vi "Shift_Value_CH0_calibration_Rev02x.vi"(0 "IN1 Shift Val1":dbl, 1 "Enable memory wright":bool, 3 "Range IN1":dbl, 4 "USB Interface Name":refnum<visa-resource-name>="COM3", 5 "Input buffer size":u32=16384, 7 "error in (no error)":errorcluster, 13 "WRITE":bool, 27 "Sign Value":dbl) -> (8 "MB address":string, 9 "MB value":u8 format="%x", 12 "UB address":string, 14 "HB address":string, 15 "error out":errorcluster, 16 "LB address":string, 17 "UB value":u8 format="%x", 19 "Data string CH0":string, 20 "IN1 shift uV":dbl, 21 "IN1 shift  HEX uV":u32 format="%x", 23 "Sign Addrss":string, 24 "HB value":u8 format="%x", 25 "LB value":u8 format="%x")   [LabVIEW 2012]
panel:
  out "LB value":string
  out "HB value":string
  out "UB value":string
  out "MB value":string
  # "1. Computes address based on the input range \"Range IN\"\n2. Take absolute values of positive and negative voltage reads in uV compares them and subtracts smaller value from the larger one. The result is devided by 2.\nIf VAL1>VAL2: ( |VAL1| - |VAL2| )/ 2"
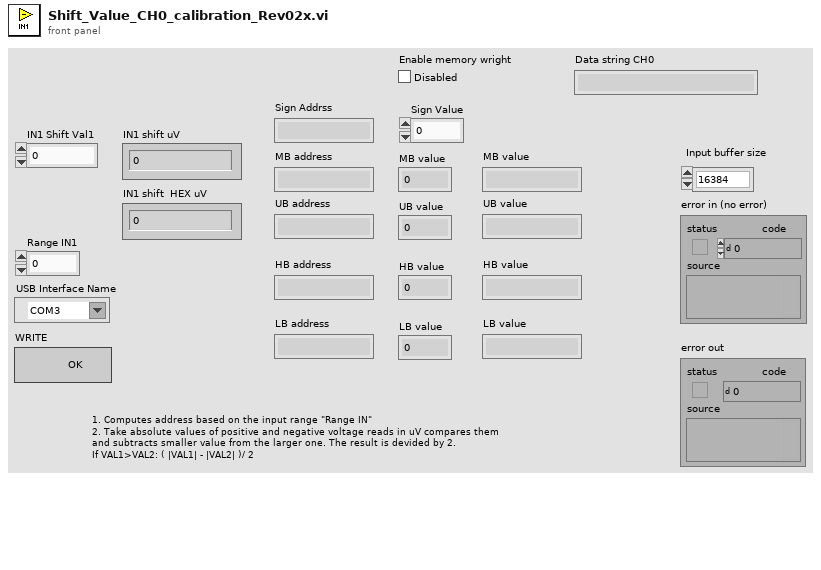
[diagram p1: front panel]
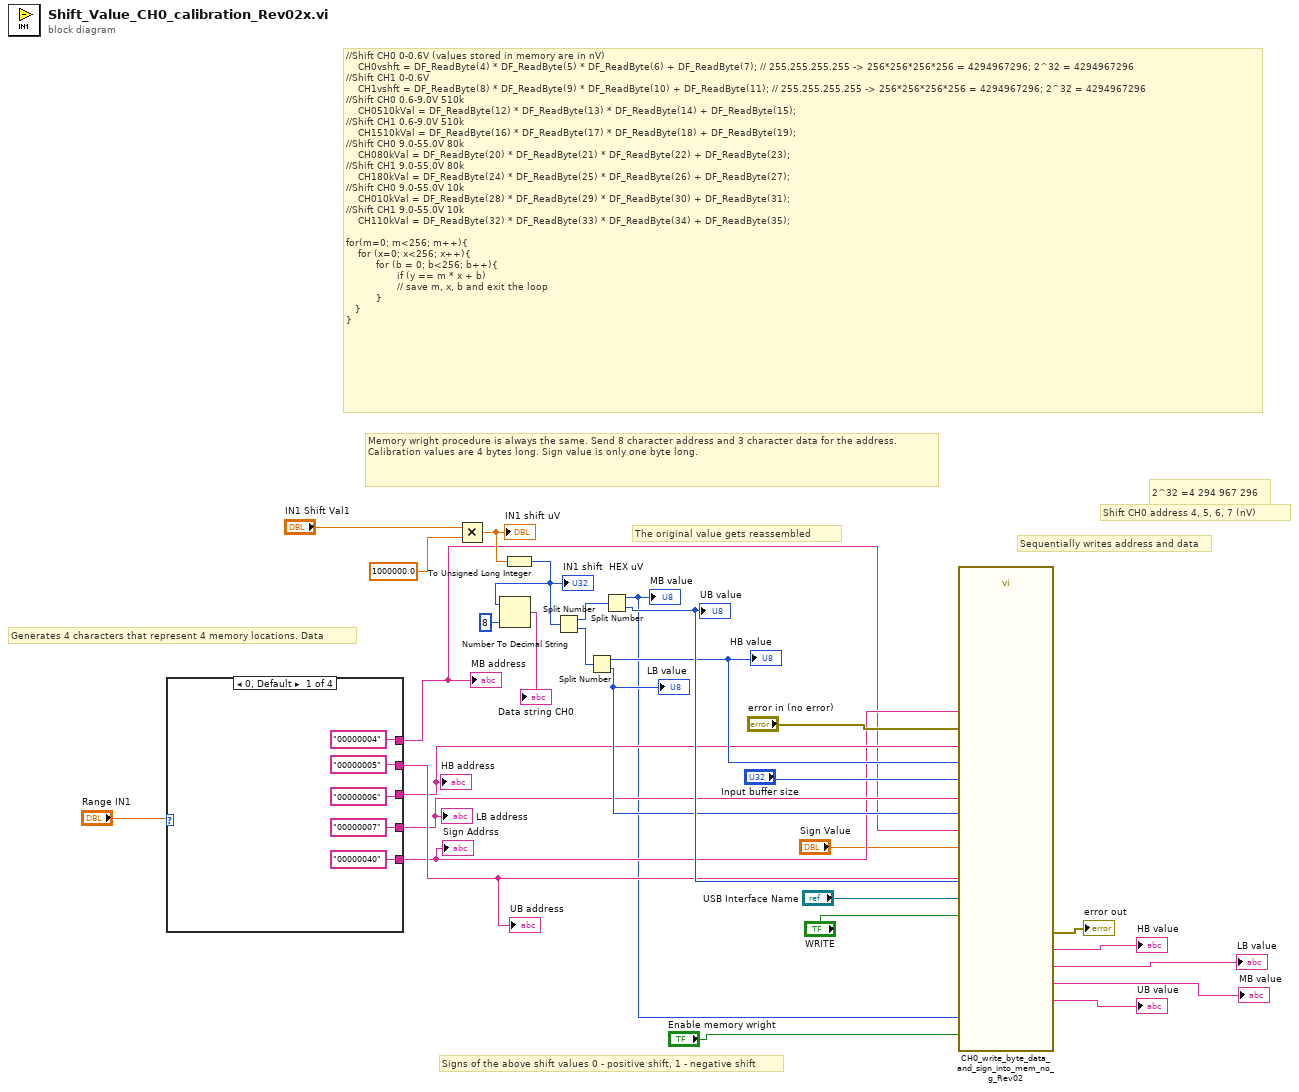
[diagram p0: block diagram]
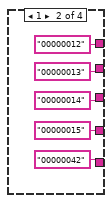
[diagram p2: hidden frame]
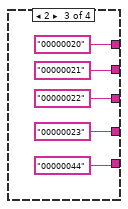
[diagram p3: hidden frame]
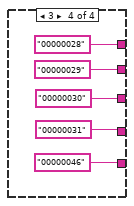
[diagram p4: hidden frame]
diagram:
  # "Shift CH0 address 4, 5, 6, 7 (nV)"
  # "Signs of the above shift values 0 - positive shift, 1 - negative shift"
  # "The original value gets reassembled"
  # "//Shift CH0 0-0.6V (values stored in memory are in nV)     \n    CH0vshft = DF_ReadByte(4) * DF_ReadByte(5) * DF_ReadByte(6) + DF_ReadByte(7); // 255.255.255.255 -> 256*256*256*256 = 4294967296; 2^32 = 4294967296\n//Shift CH1 0-0.6V\n    CH1vshft = DF_ReadByte(8) * DF_ReadByte(9) * DF_ReadByte(10) + DF_ReadByte(11); // 255.255.255.255 -> 256*256*256*256 = 4294967296; 2^32 = 4294967296\n//Shift CH0 0.6-9.0V 510k\n    CH0510kVal = DF_ReadByte(12) * DF_ReadByte(13) * DF_ReadByte(14) + DF_ReadByte(15);\n//Shift CH1 0.6-9.0V 510k\n    CH1510kVal = DF_ReadByte(16) * DF_ReadByte(17) * DF_ReadByte(18) + DF_ReadByte(19);\n//Shift CH0 9.0-55.0V 80k            \n    CH080kVal = DF_ReadByte(20) * DF_ReadByte(21) * DF_ReadByte(22) + DF_ReadByte(23);\n//Shift CH1 9.0-55.0V 80k\n    CH180kVal = DF_ReadByte(24) * DF_ReadByte(25) * DF_ReadByte(26) + DF_ReadByte(27);\n//Shift CH0 9.0-55.0V 10k\n    CH010kVal = DF_ReadByte(28) * DF_ReadByte(29) * DF_ReadByte(30) + DF_ReadByte(31);\n//Shift CH1 9.0-55.0V 10k\n    CH110kVal = DF_ReadByte(32) * DF_ReadByte(33) * DF_ReadByte(34) + DF_ReadByte(35);\n\nfor(m=0; m<256; m++){\n    for (x=0; x<256; x++){\n          for (b = 0; b<256; b++){\n                 if (y == m * x + b)\n                 // save m, x, b and exit the loop\n          }\n   }\n}"
  # "Sequentially writes address and data"
  # "Memory wright procedure is always the same. Send 8 character address and 3 character data for the address.\nCalibration values are 4 bytes long. Sign value is only one byte long."
  # "2^32 =4 294 967 296"
  # "Generates 4 characters that represent 4 memory locations. Data"
  n1 = case shown="0, Default" "Range IN1" {
    tunnel: ["00000004" "00000012" "00000020" "00000028"] -> w7
    tunnel: ["00000005" "00000013" "00000021" "00000029"] -> w19
    tunnel: ["00000006" "00000014" "00000022" "00000030"] -> w18
    tunnel: ["00000007" "00000015" "00000023" "00000031"] -> w16
    tunnel: ["00000040" "00000042" "00000044" "00000046"] -> w10
    frame 0, Default {
    }
    frame 1 {
    }
    frame 2 {
    }
    frame 3 {
    }
  }
  "MB address" <- w7
  "UB address" <- w19
  "HB address" <- w18
  "LB address" <- w16
  "Sign Addrss" <- w10
  n2 = Multiply(x="IN1 Shift Val1", y=1000000.0) -> (x*y=w8:dbl)
  "IN1 shift uV" <- w8
  n3 = To Unsigned Long Integer(number=w8) -> (unsigned 32bit integer=w3:u32)
  "IN1 shift  HEX uV" <- w3
  n4 = Number To Decimal String(number=w3, width (-)=8) -> (decimal integer string=→"Data string CH0":string)
  n5 = Split Number(x=w3) -> (hi(x)=w28:u16, lo(x)=w27:u16)
  n6 = Split Number(x=w27) -> (hi(x)=w21:u8, lo(x)=w20:u8)
  "HB value" <- w21
  "LB value" <- w20
  n7 = Split Number(x=w28) -> (hi(x)=w5:u8, lo(x)=w22:u8)
  "MB value" <- w5
  "UB value" <- w22
  n8 = call "CH0_write_byte_data_and_sign_into_mem_no_g_Rev02.vi"("MB data"=w5, "UB data"=w22, "Sign addrss 8 byte"=w10, "USB Interface Name"="USB Interface Name", "HB data"=w21, "LB data"=w20, "MB addrss 8 byte"=w7, "HB addrss 8 byte"=w18, "Sign data 3 byte"="Sign Value", "WRITE DATA"="WRITE", "Input buffer size"="Input buffer size", "LB addrss 8 byte"=w16, "UB addrss 8 byte"=w19, "error in (no error)"="error in (no error)", "Enable memory wright"="Enable memory wright") -> ("MB data 3 byte"=→"MB value":string, "UB data 3 byte"=→"UB value":string, "error out"=→"error out":errorcluster, "HB data 3 byte"=→"HB value":string, "LB data 3 byte"=→"LB value":string)
